vi "subvi_percent.vi"(4 "Function":enum16{"+", "-", "/", "*", "sqrt", "%"}(ring), 8 "Input in":dbl, 9 "Input 1":dbl) -> (3 "Answer":dbl)   [LabVIEW 2020]
panel:
  # "Calculator A:\n\n90 [+] 10 [%] = 99\t      calculates as: \t90 + (10% of 90) = 99\n90 [-] 10 [%] = 81\t      calculates as: \t90 - (10% of 90) = 81\n90 [x] 10 [%] = 9\t      calculates as: \t90 x (0.1) = 9\n90 [/] 10 [%] = 900\t      calculates as: \t90 / (0.1) = 900\n10 [%] = 0\t      calculates as: \tcalculator does not process\n\nNotice that the [x] and [/] operators cause the percent button to function differently than the [+] and [-] operators.\nFor the [+] and [-] operators, the calculator sees the 10 [%] as 10% of 90 which is equal to 9.\nFor the [x] and [/] operators, the calculator sees the 10 [%] as 10/100 which is equal to 0.1"
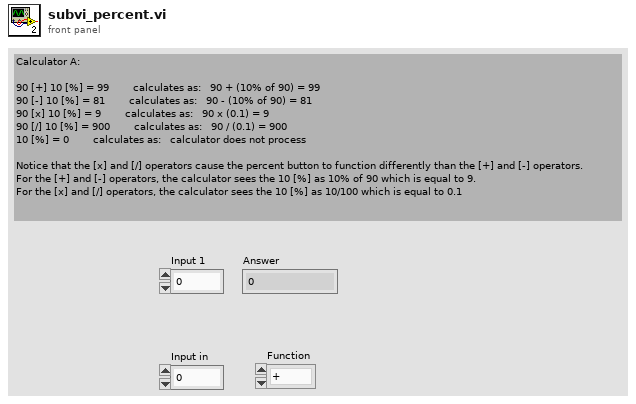
[diagram p1: front panel]
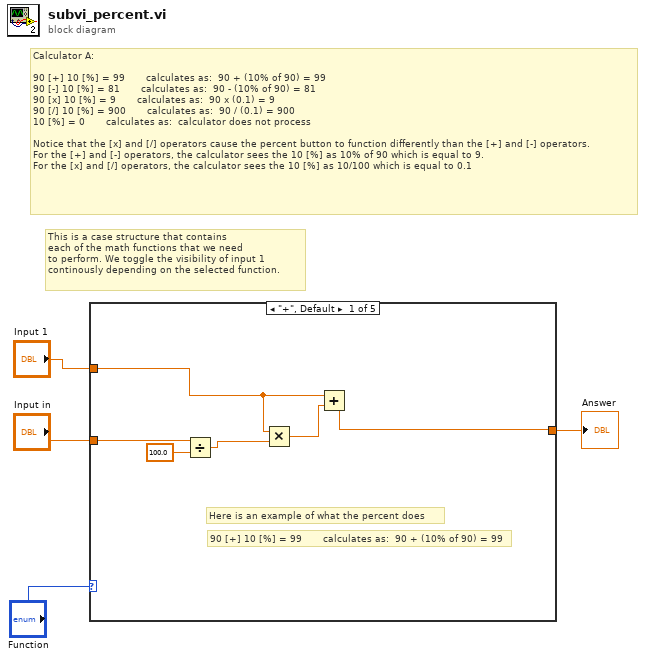
[diagram p0: block diagram]
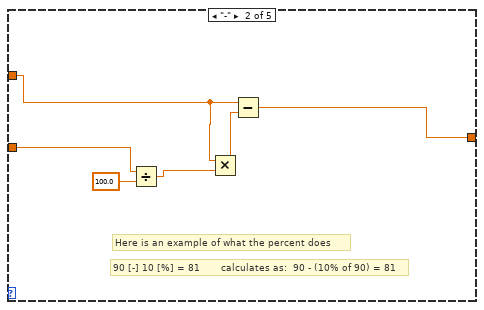
[diagram p2: hidden frame]
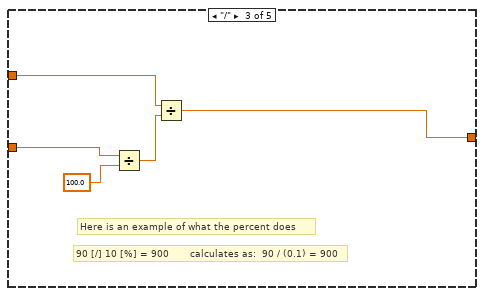
[diagram p3: hidden frame]
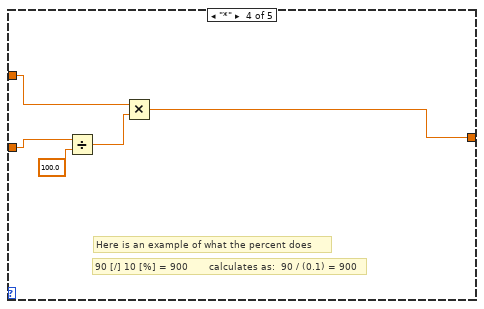
[diagram p4: hidden frame]
diagram:
  # "Calculator A:\n\n90 [+] 10 [%] = 99\t      calculates as: \t90 + (10% of 90) = 99\n90 [-] 10 [%] = 81\t      calculates as: \t90 - (10% of 90) = 81\n90 [x] 10 [%] = 9\t      calculates as: \t90 x (0.1) = 9\n90 [/] 10 [%] = 900\t      calculates as: \t90 / (0.1) = 900\n10 [%] = 0\t      calculates as: \tcalculator does not process\n\nNotice that the [x] and [/] operators cause the percent button to function differently than the [+] and [-] operators.\nFor the [+] and [-] operators, the calculator sees the 10 [%] as 10% of 90 which is equal to 9.\nFor the [x] and [/] operators, the calculator sees the 10 [%] as 10/100 which is equal to 0.1"
  # "This is a case structure that contains\neach of the math functions that we need \nto perform. We toggle the visibility of input 1\ncontinously depending on the selected function."
  n1 = case shown="\"+\", Default" "Function" {
    tunnel: "Input 1" -> [w6 w13 w21 w26 _]
    tunnel: "Input in" -> [w9 w11 w19 w24 w27]
    tunnel: [w10 w16 w20 w25 w27] -> w3
    frame "+", Default {
      # "Here is an example of what the percent does"
      # "90 [+] 10 [%] = 99\t      calculates as: \t90 + (10% of 90) = 99"
      n2 = Divide(x=w9, y=100.0) -> (x/y=w7:dbl)
      n3 = Multiply(x=w6, y=w7) -> (x*y=w5:dbl)
      n4 = Add(x=w6, y=w5) -> (x+y=w10:dbl)
    }
    frame "-" {
      # "Here is an example of what the percent does"
      # "90 [-] 10 [%] = 81\t      calculates as: \t90 - (10% of 90) = 81"
      n5 = Divide(x=w11, y=100.0) -> (x/y=w14:dbl)
      n6 = Multiply(x=w13, y=w14) -> (x*y=w12:dbl)
      n7 = Subtract(x=w13, y=w12) -> (x-y=w16:dbl)
    }
    frame "/" {
      # "Here is an example of what the percent does"
      # "90 [/] 10 [%] = 900\t      calculates as: \t90 / (0.1) = 900"
      n8 = Divide(x=w19, y=100.0) -> (x/y=w17:dbl)
      n9 = Divide(x=w21, y=w17) -> (x/y=w20:dbl)
    }
    frame "*" {
      # "90 [/] 10 [%] = 900\t      calculates as: \t90 / (0.1) = 900"
      # "Here is an example of what the percent does"
      n10 = Divide(x=w24, y=100.0) -> (x/y=w22:dbl)
      n11 = Multiply(x=w26, y=w22) -> (x*y=w25:dbl)
    }
    frame "sqrt" {
      # "We dont do anything here."
    }
  }
  "Answer" <- w3
